vi "test Deploy Scripted System Definition.vi"(8 "error in (no error)":errorcluster, 11 "TestCase in":refnum<class "SLSC Switch Scripting System Tests.lvclass">=refnum) -> (0 "error out":errorcluster, 3 "TestCase out":refnum<class "SLSC Switch Scripting System Tests.lvclass">)   [LabVIEW 2017, in "SLSC Switch Scripting System Tests.lvclass"]
uses:
  SLSC Switch Scripting System Tests.lvclass
  <vilib>/addons/_JKI Toolkits/VI Tester/TestCase.llb/TestCase.lvclass
  niveristand-custom-device-testing-tools/VeriStandTestCase/VeriStandTestCase.lvclass
  NationalInstruments.VeriStand.SystemDefinitionAPI
  C:/Users/nitest/Desktop/Git/niveristand-custom-device-testing-tools/VeriStandTestCase/VeriStandTestCase.lvclass
  C:/Program Files (x86)/National Instruments/LabVIEW 2017/vi.lib/addons/_JKI Toolkits/VI Tester/TestCase.llb/TestCase.lvclass
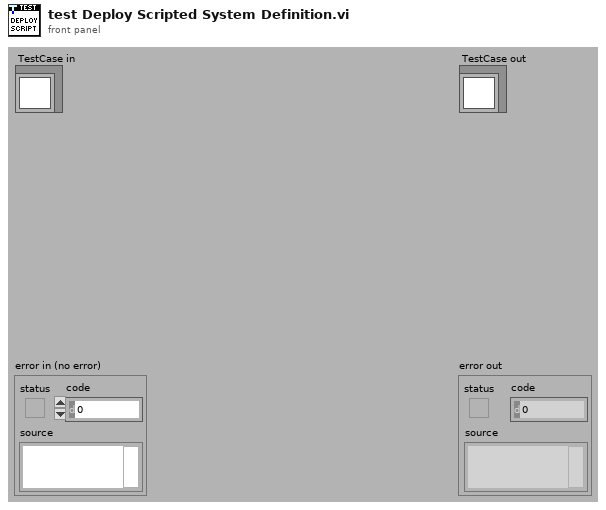
[diagram p1: front panel]
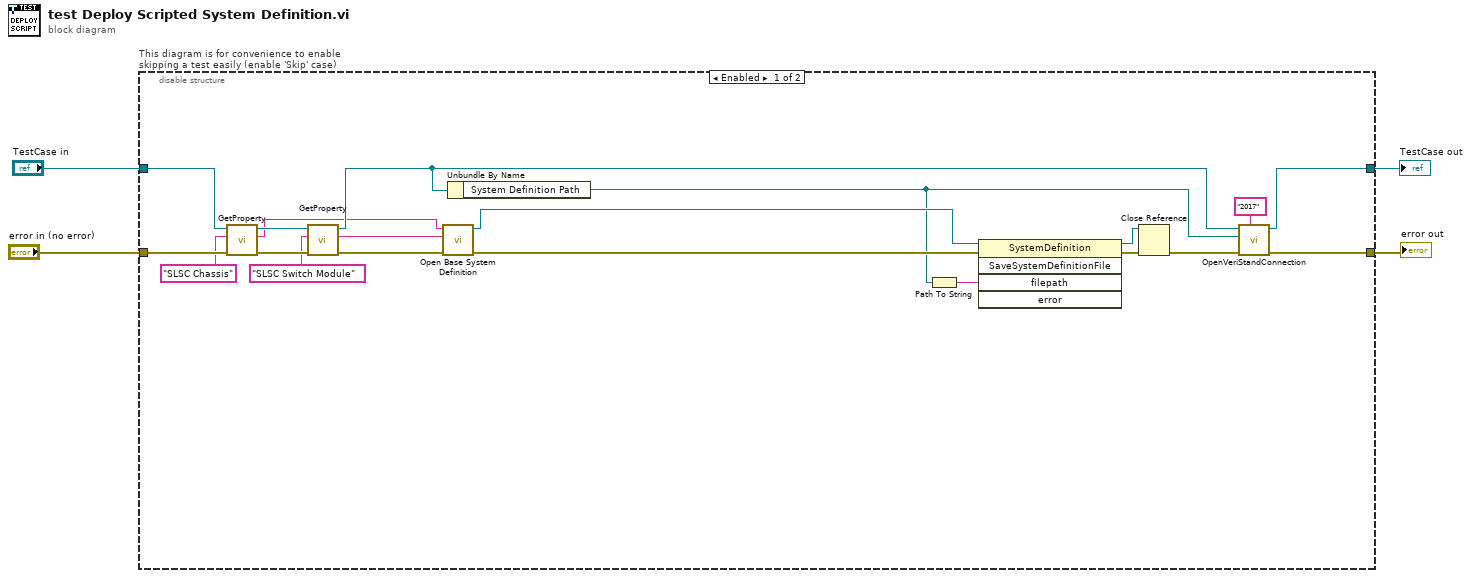
[diagram p0: block diagram]
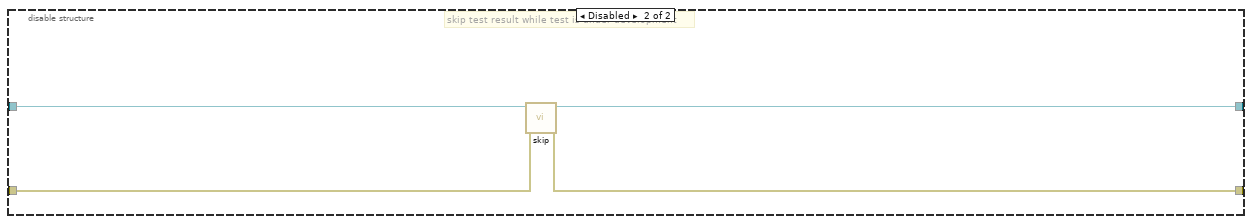
[diagram p2: hidden frame]
diagram:
  n1 = disable-structure "This diagram is for convenience to enable skipping a test easily (enable 'Skip' case)" shown="Enabled" {
    disable-tunnel: "TestCase in" -> [w13 w28]
    disable-tunnel: [w24 w26] -> w1
    disable-tunnel: [w23 w27] -> w3
    disable-tunnel: "error in (no error)" -> [w14 w25]
    frame Enabled {
      n2 = call "GetProperty.vi"("error in (no error)"=w14, "key"="SLSC Chassis", "VeriStandTestCase in"=w13) -> ("error out"=w11:errorcluster, "value"=w6:string, "VeriStandTestCase out"=w9:refnum<class "SLSC Switch Scripting System Tests.lvclass">)  [unwired: 6 in]
      n3 = call "GetProperty.vi"("error in (no error)"=w11, "key"="SLSC Switch Module", "VeriStandTestCase in"=w9) -> ("error out"=w10:errorcluster, "value"=w5:string, "VeriStandTestCase out"=w8:refnum<class "SLSC Switch Scripting System Tests.lvclass">)  [unwired: 6 in]
      n4 = call "Open Base System Definition.vi"("error in (no error)"=w10, "SLSC Switch Module"=w5, "SLSC Chassis Name or IP"=w6) -> ("error out"=w22:errorcluster, "SystemDefinition"=w21:refnum<k24>)  [unwired: 6 in, 1 out]
      n5 = Unbundle By Name(w8) -> ("System Definition Path"=w17:path)
      n6 = Path To String(path=w17) -> (string=w18:string)
      n7 = invoke class="SystemDefinition" method="SaveSystemDefinitionFile"(reference=w21, error in=w22, "filepath"=w18) -> (reference out=w19:refnum<k24>, error out=w20:errorcluster)  [unwired: 2 in, 3 out]
      n8 = Close Reference(reference=w19, error in (no error)=w20) -> (error out=w15:errorcluster)
      n9 = call-dynamic "OpenVeriStandConnection.vi"("Minimum VeriStand Version (2016)"="2017" ("Minimum VeriStand Version (2015)"), "error in (no error)"=w15, "System Definition File"=w17, "VeriStand Test Case in"=w8) -> ("error out"=w23:errorcluster, "VeriStand Test Case out"=w24:refnum<class "SLSC Switch Scripting System Tests.lvclass">)  [unwired: 5 in, 1 out]
    }
    frame Disabled {
      # "skip test result while test is under development"
      n10 = call <vilib>:"skip.vi"("error in (no error)"=w25, "TestCase in"=w28) -> ("error out"=w27:errorcluster, "TestCase out"=w26:refnum<class "SLSC Switch Scripting System Tests.lvclass">)  [unwired: 8 in]
    }
  }
  "error out" <- w3
  "TestCase out" <- w1
